vi "save_array_to_image.vi"(10 "Image\ndata":i16[][](array[numeric])) -> ()   [LabVIEW 2011]
uses:
  Action Items.ctl
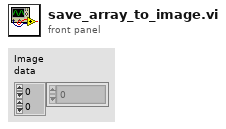
[diagram p1: front panel]
types:
  T1 = typedef "Action Items.ctl" = enum16{"Initialize", "Get"}
  T2 = typedef "Image Type" = u32
  T3 = cluster{"Rows Per Strip":i32, "Photometric":i32, "Compression Type":i32}
  T4 = cluster{"Path":string, "Filestemname":string, "Filestemname incl path":string, "Filename incl path":string}
  T5 = typedef "IMAQ Image.ctl" = refnum<image>
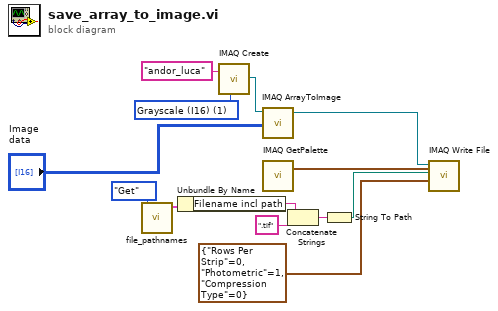
[diagram p0: block diagram]
diagram:
  w7 = T2 1 items=["Grayscale (U8)", "Grayscale (I16)", "Grayscale (SGL)", "Complex (CSG)", "RGB (U32)", "HSL (U32)", "RGB (U64)", "Grayscale (U16)"] ("Image Type")
  n1 = call "file_pathnames.vi"("Action"=Action_Items."Get") -> ("File-path\n-names"=w4:T4)  [unwired: 10 in]
  n2 = Unbundle By Name(w4) -> ("Filename incl path"=w1:string)
  n3 = call "IMAQ Create"("Image Name"="andor_luca", "Image Type"=w7) -> ("New Image"=w9:T5)  [unwired: 3 in, 1 out]
  n4 = call "IMAQ ArrayToImage"("Image Pixels (I16)"="Image\ndata", "Image"=w9) -> ("Image Out"=w13:T5)  [unwired: 8 in, 1 out]
  n5 = call "IMAQ GetPalette"() -> ("Color Palette"=w11:cluster{"Red":u8, "Green":u8, "Blue":u8}[])  [unwired: 5 in, 1 out]
  n6 = Concatenate Strings(w1, ".tif" ("string")) -> (w2:string)
  n7 = String To Path(string=w2) -> (path=w10:path)
  n8 = call-poly "IMAQ Write File"("Color Palette"=w11, "TIFF Options"=T3 {"Rows Per Strip"=0, "Photometric"=1, "Compression Type"=0}, "File Path"=w10, "Image"=w13) -> ()  [unwired: 6 in, 2 out]
